vi "Get Legend Axis.vi"(8 "error in (no error)":errorcluster, 11 "3D Plot in":refnum<class "3D Plot.lvclass">) -> (0 "error out":errorcluster, 1 "Active Axis":enum16{"X-axis", "Y-axis", "Z-axis"}(ring)=enum."Z-axis", 3 "3D Plot out":refnum<class "3D Plot.lvclass">)   [LabVIEW 2017, in "3D Plot.lvclass"]
uses:
  <vilib>/Math Plots/3D Math Plots/3D Plot/3D Plot/3D Plot.lvclass
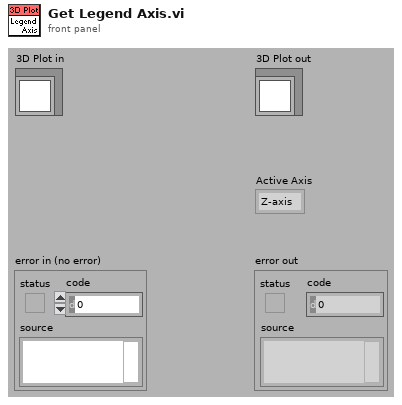
[diagram p1: front panel]
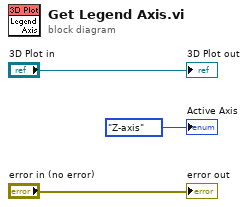
[diagram p0: block diagram]
diagram:
  "error out" <- "error in (no error)"
  "3D Plot out" <- "3D Plot in"
  "Active Axis" <- enum16{"X-axis", "Y-axis", "Z-axis"}."Z-axis" ("Active Axis")
